vi "Control_Motor_Galil_Hz.vi"() -> ()   [LabVIEW 2015]
uses:
  <vilib>/Instr/_visa.llb/VISA Configure Serial Port (Instr).vi
  <vilib>/regexp/Match Regular Expression.xnode
panel:
  in  "Velocidad":dbl=1.0 format="%#_13g"
  in  "Instrucciones":bool
  in  "No. de Ciclos":dbl=10.0 format="%#_13g"
  in  "Frecuencia":dbl=1.0 format="%#_13g"
  in  "Amplitud":dbl=0.5 format="%#_13g"
  in  "waves 2":bool
  in  "time to save":dbl=0.1
  out "x = y?":bool
  out "GUARDAR":bool
  out "TORQUE":dbl
  out "carga":bool
  out "Boolean 3":bool
  out "whole match":string
  out "size(s)":i32
  out "element":string
  out "x = y? 2":bool
  out "VARIABLE Y":dbl format="%.2f"
  out "VARIABLE X":dbl format="%.2f"
  in  "Combo Box 2":string(combo)="DESPLAZAMIENTO [mm]"
  in  "Combo Box":string(combo)="TIEMPO [s]"
  out "XY Graph":cluster{"TIME SEC":dbl[], "ATT":dbl[]}(graph)
  out "TIME SEC":dbl[](array[numeric]) format="%.2f"
  out "ADD":dbl[](array[numeric]) format="%.2f"
  out "ATT":dbl[](array[numeric]) format="%.2f"
  out "AT":dbl[](array[numeric])
  out "AD":dbl[](array[numeric])
  out "x/y":dbl
  out "result string 2":string
  out "after match":string
  out "result string":string
  out "before match":string
  out "Boolean 2":bool
  out "tiempo [min]":ext
  out "path":path
  out "desplazamiento":dbl format="%.2f"
  out "torque":dbl format="%.2f"
  in  "detener":bool
  in  "VISA resource name":refnum<visa-resource-name>="COM14"
  in  "stop":bool
  in  "bajar":bool
  out "String 2":string
  in  "stop 2":bool
  in  "Filename":path=path "Datos_Motor_Dyn"
  in  "subir":bool
  in  "waves":bool
  in  "Movimiento manual":bool
  out "read buffer":string
  out "return count READ":u32
  out "VARIABLE":string
  out "return count 1":u32
  in  "POSICION":dbl
  out "PULSOS":dbl
  in  "code":string
  out "initialized array":string[](array[string])
  # "EJE X"
  # "EJE Y"
  # "Tiempo adquisición"
  # "Guardando"
  # "[mm/s]"
  # "[mm]"
  # "[Hz]"
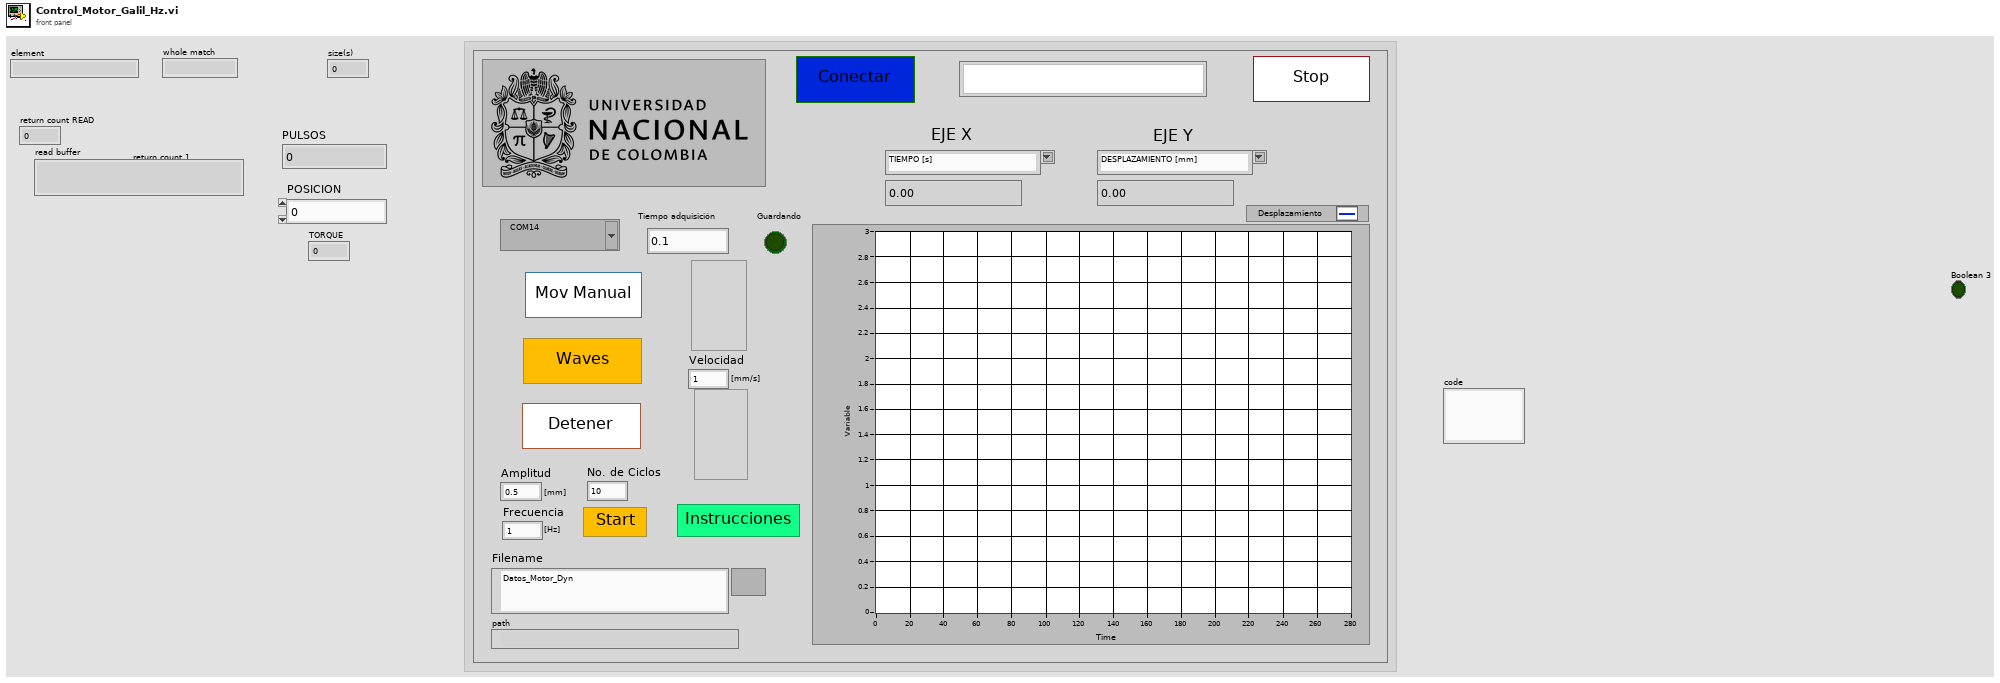
[diagram p1: front panel]
types:
  T1 = enum16{"open", "open or create", "create or replace", "create", "open (read-only)"}
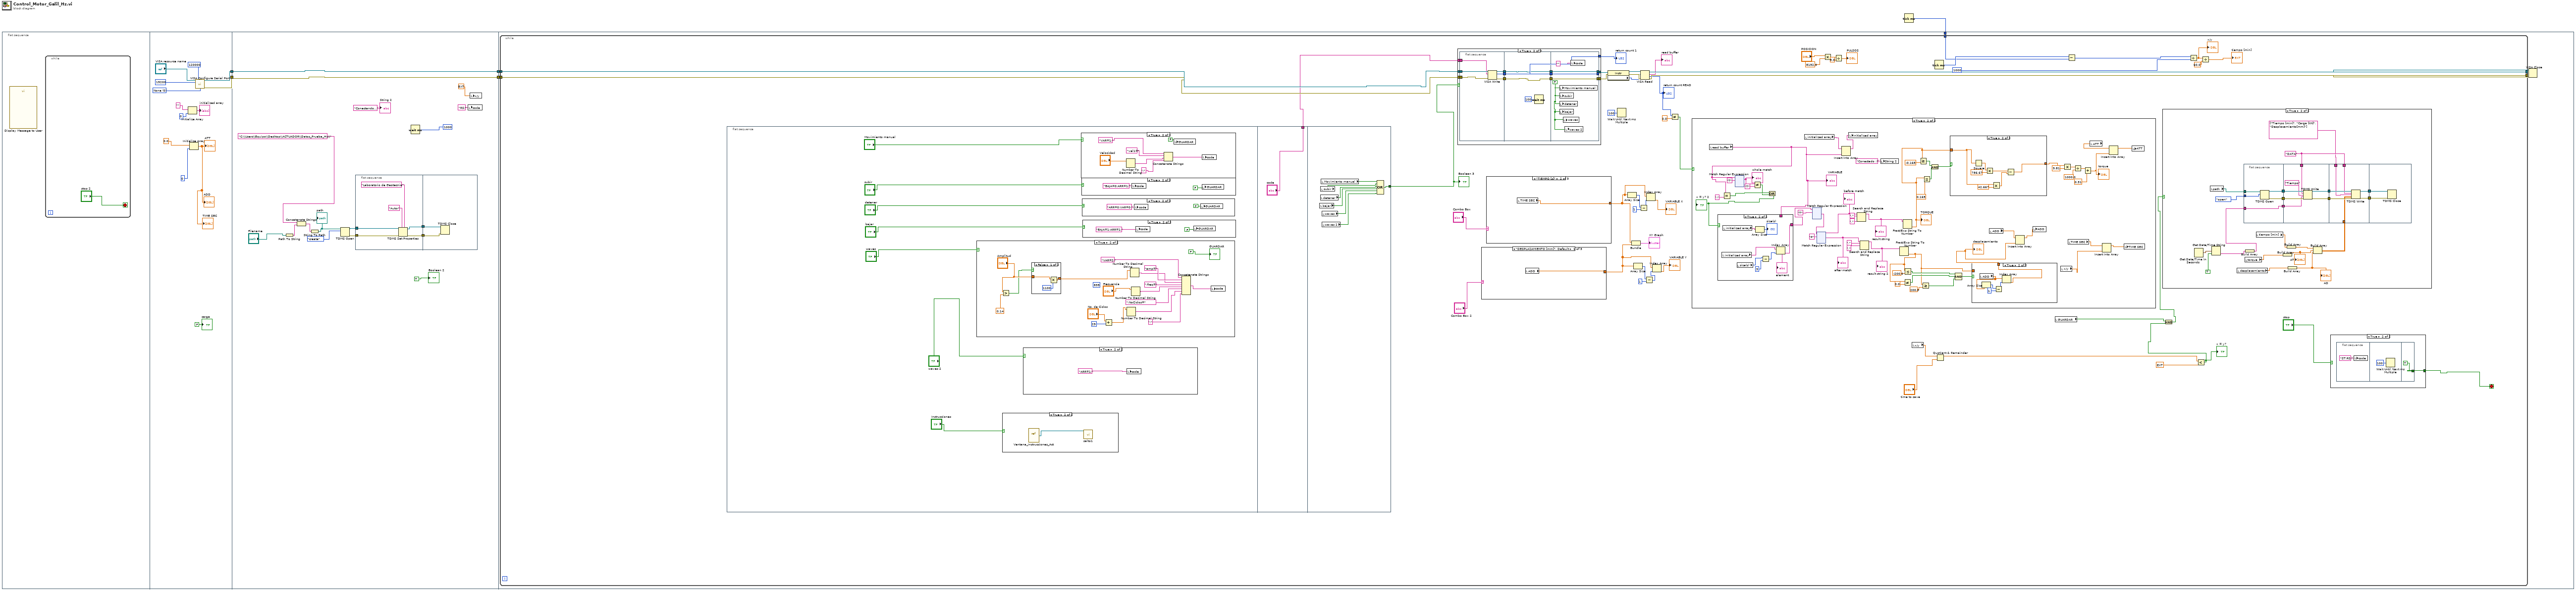
[diagram p0: block diagram]
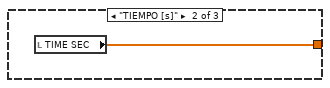
[diagram p3: hidden frame]
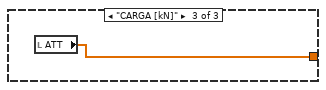
[diagram p4: hidden frame]
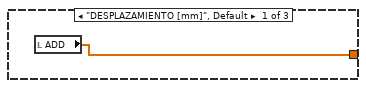
[diagram p5: hidden frame]
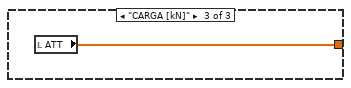
[diagram p6: hidden frame]
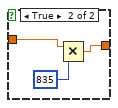
[diagram p11: hidden frame]
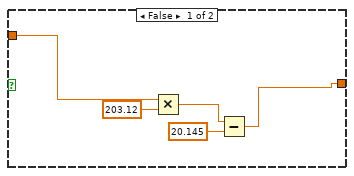
[diagram p19: hidden frame]
diagram:
  n1 = flat-sequence {
    tunnel: [w13] -> w5
    tunnel: [w12] -> w4
    tunnel: [w35] -> w3
    tunnel: [w34] -> w2
    tunnel: w5 -> [w35]
    tunnel: w4 -> [w34]
    tunnel: w3 -> [w49]
    tunnel: w2 -> [w48]
    tunnel: w1 -> [w45]
    frame #0 {
      n2 = call "Display Message to User"() -> ()  [unwired: 10 in, 2 out]
      n3 = while {
        stop <- "stop 2" stop-if-true
      }
    }
    frame #1 {
      w19 = u16 0 items=["None", "XON/XOFF", "RTS/CTS", "XON/XOFF & RTS/CTS", "DTR/DSR", "XON/XOFF & DTR/DSR"] ("flow control (0:none)")
      n4 = Initialize Array("", 0 ("dimension size")) -> (→"initialized array":string[])
      n5 = Initialize Array(0.0, 0 ("dimension size")) -> (→"ATT" →"ADD" →"TIME SEC":dbl[])
      n6 = call-poly "VISA Configure Serial Port"("VISA resource name"="VISA resource name", "timeout (10sec)"=u32 120000, "baud rate (9600)"=u32 19200, "flow control (0:none)"=w19) -> ("VISA resource name out"=w13:refnum<visa-resource-name>, "error out"=w12:errorcluster)  [unwired: 10 in]
      "carga" <- FALSE ("carga")
    }
    frame #2 {
      n7 = Path To String(path="Filename") -> (string=w31:string)
      n8 = Concatenate Strings("C:\\Users\\Equipo\\Desktop\\ACTUADOR\\Datos_Prueba_Hz\\", w31) -> (w30:string)
      n9 = String To Path(string=w30) -> (path=w28:path)
      "path" <- w28
      n10 = TDMS Open(10:T1."create" ("operation (0:open)"), 11:w28) -> (0:w24:errorcluster, 3:w25:refnum<k34>)  [unwired: 5 in]
      n11 = flat-sequence {
        tunnel: [w40] -> w33
        tunnel: [w39] -> w32
        tunnel: w25 -> [w38]
        tunnel: w24 -> [w37]
        tunnel: w33 -> [w44]
        tunnel: w32 -> [w43]
        frame #0 {
          n12 = TDMS Set Properties(5:"Laboratorio de Geotecnia" ("property name"), 7:"Autor" ("property name"), 8:w37, 11:w38) -> (0:w39:errorcluster, 3:w40:refnum<k34>)  [unwired: 2 in, 2 out]
        }
        frame #1 {
          n13 = TDMS Close(8:w43, 11:w44) -> ()  [unwired: 2 out]
        }
      }
      n14 = Wait (ms)(milliseconds to wait=u32 1000) -> ()  [unwired: 1 out]
      n15 = local write "code"("RS;" ("code")) -> ()
      n16 = local write "x/y"(ext 0.0 ("x-y*floor(x/y)")) -> ()
      "String 2" <- "Conectando..." ("String 2")
      "Boolean 2" <- TRUE
    }
    frame #3 {
      n17 = while {
        tunnel: w49 -> [w89]
        tunnel: w48 -> [w88]
        tunnel: [w96] -> w47
        tunnel: [w95] -> w46
        tunnel: w45 -> [w72]
        stop <- w58 stop-if-true
        n18 = flat-sequence {
          tunnel: ["code"] -> w79
          tunnel: [w202] -> w80
          frame #0 {
            n19 = case shown="True" "waves" {
              frame False {
              }
              frame True {
                (unwired) 835
                n20 = Greater?(x="Amplitud", y=0.14) -> (0:w163:bool)
                n21 = case shown="False" w163 {
                  tunnel: [w181 w185] -> w166
                  tunnel: "Amplitud" -> [w182 w184]
                  frame False {
                    n22 = Multiply(x=w182, y=1100) -> (x*y=w181:dbl)
                  }
                  frame True {
                    n23 = Multiply(x=w184, y=835) -> (x*y=w185:dbl)
                  }
                }
                n24 = Add(x="No. de Ciclos", y=29) -> (x+y=w171:dbl)
                n25 = Number To Decimal String(number=w171) -> (decimal integer string=w173:string)  [unwired: 1 in]
                n26 = Number To Decimal String(number=w166) -> (decimal integer string=w177:string)  [unwired: 1 in]
                n27 = Number To Decimal String(number="Frecuencia") -> (decimal integer string=w167:string)  [unwired: 1 in]
                n28 = Concatenate Strings("VAR=2;" ("code"), "amp=", w177, ";freq=", w167, ";NoCiclos=", w173, ";") -> (w174:string)
                n29 = local write "code"(w174) -> ()
                "GUARDAR" <- FALSE
              }
            }
            n30 = case shown="True" "Instrucciones" {
              frame False {
              }
              frame True {
                n31 = vi-ref "Ventana_Instrucciones_Act.vi"() -> (w161:refnum<vi>)
                n32 = call "salto1.vi"("reference"=w161) -> ()  [unwired: 15 in]
              }
            }
            n33 = case shown="True" "waves 2" {
              frame False {
              }
              frame True {
                n34 = local write "code"("ARR=1;" ("code")) -> ()
              }
            }
            n35 = case shown="True" "Movimiento manual" {
              frame False {
              }
              frame True {
                n36 = Number To Decimal String(number="Velocidad") -> (decimal integer string=w194:string)  [unwired: 1 in]
                n37 = Concatenate Strings("VAR=1;" ("code"), "vel1=", w194, ";") -> (w197:string)
                n38 = local write "GUARDAR"(FALSE) -> ()
                n39 = local write "code"(w197) -> ()
              }
            }
            n40 = case shown="True" "subir" {
              frame False {
              }
              frame True {
                n41 = local write "code"("BAJA=0;ARR=1;" ("code")) -> ()
                n42 = local write "GUARDAR"(FALSE ("GUARDAR")) -> ()
              }
            }
            n43 = case shown="True" "detener" {
              frame False {
              }
              frame True {
                n44 = local write "code"("ARR=0;VAR=0;" ("code")) -> ()
                n45 = local write "GUARDAR"(FALSE ("GUARDAR")) -> ()
              }
            }
            n46 = case shown="True" "bajar" {
              frame False {
              }
              frame True {
                n47 = local write "code"("BAJA=1;ARR=1;" ("code")) -> ()
                n48 = local write "GUARDAR"(FALSE ("GUARDAR")) -> ()
              }
            }
          }
          frame #1 {
          }
          frame #2 {
            n49 = local read "bajar"() -> (w206:bool)
            n50 = local read "detener"() -> (w205:bool)
            n51 = local read "subir"() -> (w204:bool)
            n52 = local read "Movimiento manual"() -> (w203:bool)
            n53 = local read "waves"() -> (w207:bool)
            n54 = local read "waves 2"() -> (w201:bool)
            n55 = Compound Arithmetic op=OR(w203, w204, w205, w206, w207, w201) -> (w202:bool)
          }
        }
        n56 = case shown="True" w80 {
          tunnel: w89 -> [w629 w638]
          tunnel: w88 -> [w628 w637]
          tunnel: [w629 w636] -> w90
          tunnel: [w628 w635] -> w100
          tunnel: w79 -> [_ w634]
          tunnel: [_ w633] -> w87
          frame False {
          }
          frame True {
            n57 = flat-sequence {
              tunnel: w638 -> [w647]
              tunnel: w637 -> [w646]
              tunnel: [w645] -> w641
              tunnel: [w644] -> w640
              tunnel: [w643] -> w639
              tunnel: w634 -> [w642]
              tunnel: w641 -> [w649]
              tunnel: w640 -> [w648]
              tunnel: w639 -> [w651]
              tunnel: [w649] -> w632
              tunnel: [w648] -> w631
              tunnel: [w651] -> w630
              tunnel: [w654] -> w633
              tunnel: [w655] -> w635
              tunnel: [w656] -> w636
              tunnel: w632 -> [w656]
              tunnel: w631 -> [w655]
              tunnel: w630 -> [w654]
              frame #0 {
                n58 = VISA Write(VISA resource name=w647, write buffer=w642, error in (no error)=w646) -> (VISA resource name out=w645:refnum<visa-resource-name>, return count=w643:u32, error out=w644:errorcluster)
              }
              frame #1 {
                n59 = Wait (ms)(milliseconds to wait=u32 100) -> ()  [unwired: 1 out]
              }
              frame #2 {
                w652 = FALSE
                n60 = local write "Movimiento manual"(w652) -> ()
                n61 = local write "subir"(w652) -> ()
                n62 = local write "detener"(w652) -> ()
                n63 = local write "bajar"(w652) -> ()
                n64 = local write "waves"(w652) -> ()
                n65 = local write "waves 2"(w652) -> ()
                n66 = local write "code"("" ("code")) -> ()
              }
            }
          }
        }
        "return count 1" <- w87
        n67 = case shown="\"DESPLAZAMIENTO [mm]\", Default" "Combo Box 2" {
          tunnel: [w105 w106 w107] -> w65
          frame "DESPLAZAMIENTO [mm]", Default {
            n68 = local read "ADD"() -> (w105:dbl[])
          }
          frame "TIEMPO [s]" {
            n69 = local read "TIME SEC"() -> (w106:dbl[])
          }
          frame "CARGA [kN]" {
            n70 = local read "ATT"() -> (w107:dbl[])
          }
        }
        n71 = case shown="\"TIEMPO [s]\"" "Combo Box" {
          tunnel: [w108 w109 w110] -> w67
          frame "DESPLAZAMIENTO [mm]", Default {
            n72 = local read "ADD"() -> (w108:dbl[])
          }
          frame "TIEMPO [s]" {
            n73 = local read "TIME SEC"() -> (w109:dbl[])
          }
          frame "CARGA [kN]" {
            n74 = local read "ATT"() -> (w110:dbl[])
          }
        }
        n75 = property class="Instr"(reference=w90, error in=w100) -> (reference out=w99:refnum<visa-resource-name>, error out=w98:errorcluster, "Serial Settings:Number of Bytes at Serial Port"=w97:u32)
        n76 = Wait Until Next ms Multiple(millisecond multiple=u32 100) -> ()  [unwired: 1 out]
        n77 = Array Size(array=w67) -> (size(s)=w61:i32)
        n78 = Bundle("ATT"=w67, "ATT"=w65) -> (→"XY Graph":cluster{"ATT":dbl[], "ATT":dbl[]})  [unwired: 1 in]
        n79 = Array Size(array=w65) -> (size(s)=w64:i32)
        n80 = Subtract(x=w61, y=1) -> (x-y=w60:i32)
        n81 = VISA Read(VISA resource name=w99, byte count=w97, error in (no error)=w98) -> (VISA resource name out=w96:refnum<visa-resource-name>, read buffer=→"read buffer":string, return count=w91:u32, error out=w95:errorcluster)
        "return count READ" <- w91
        n82 = Subtract(x=w64, y=1) -> (x-y=w63:i32)
        n83 = Index Array(array=w67, index=w60) -> (element=→"VARIABLE X":dbl)
        n84 = Index Array(array=w65, index=w63) -> (element=→"VARIABLE Y":dbl)
        n85 = Not Equal?(x=w91, y=0.0) -> (x != y?=w93:bool)
        n86 = case shown="True" w93 {
          frame False {
          }
          frame True {
            n87 = local read "read buffer"() -> (w226:string)
            "VARIABLE" <- w226
            n88 = Equal?(x=w226, y=":") -> (x = y?=w224:bool)
            n89 = xnode "Match Regular Expression"("input string"=w226, "regular expression"="T") -> ("whole match"=w222:string)  [unwired: 4 in, 4 out]
            "whole match" <- w222
            n90 = Not Equal?(x=w222, y="T") -> (x != y?=w220:bool)
            n91 = Or(x=w224, y=w220) -> (x .or. y?=w223:bool)
            "x = y? 2" <- w223
            n92 = case shown="True" w223 {
              tunnel: [w380 w387] -> w227
              tunnel: w226 -> [w380 _]
              frame False {
              }
              frame True {
                n93 = local read "initialized array"() -> (w386:string[])
                n94 = local read "initialized array"() -> (w385:string[])
                n95 = local read "size(s)"() -> (w383:i32)
                n96 = Array Size(array=w385) -> (size(s)=→"size(s)":i32)
                n97 = Subtract(x=w383, y=3) -> (x-y=w381:i32)
                n98 = Index Array(array=w386, index=w381) -> (element=w387:string)
                "element" <- w387
              }
            }
            n99 = local read "initialized array"() -> (w258:string[])
            n100 = xnode "Match Regular Expression"("input string"=w227, "regular expression"="T") -> ("after match"=w254:string)  [unwired: 4 in, 4 out]
            n101 = xnode "Match Regular Expression"("input string"=w254, "regular expression"="P") -> ("before match"=w253:string, "after match"=w247:string)  [unwired: 4 in, 3 out]
            "before match" <- w253
            "after match" <- w247
            n102 = Insert Into Array(array=w258, new element=w226) -> (w259:string[])  [unwired: 1 in]
            n103 = local write "initialized array"(w259) -> ()
            n104 = Search and Replace String(input string=w253, search string=".", replace string="," ("replace string (\"\")")) -> (result string=w250:string)  [unwired: 5 in, 3 out]
            "result string" <- w250
            n105 = Search and Replace String(input string=w247, search string=".", replace string="," ("replace string (\"\")")) -> (result string=w248:string)  [unwired: 5 in, 3 out]
            "result string 2" <- w248
            n106 = local write "String 2"("Conectado :)" ("String 2")) -> ()
            n107 = Fract/Exp String To Number(string=w248) -> (number=w213:dbl)  [unwired: 3 in, 1 out]
            n108 = Fract/Exp String To Number(string=w250) -> (number=w233:dbl)  [unwired: 3 in, 1 out]
            "TORQUE" <- w233
            n109 = Not Equal?(x=w213, y=0.0) -> (x != y?=w217:bool)
            n110 = Less Or Equal?(x=w213, y=-200.0) -> (x <= y?=w218:bool)
            n111 = Greater Or Equal?(x=w233, y=-0.165) -> (x >= y?=w236:bool)
            n112 = Greater Or Equal?(x=w213, y=200.0) -> (x >= y?=w216:bool)
            n113 = Less Or Equal?(x=w233, y=0.165) -> (x <= y?=w237:bool)
            n114 = And(x=w236, y=w237) -> (x .and. y?=w238:bool)
            n115 = case shown="True" w238 {
              tunnel: w233 -> [w392 w396]
              tunnel: [w388 w393] -> w232
              frame False {
                n116 = Multiply(x=w392, y=203.12) -> (x*y=w390:dbl)
                n117 = Subtract(x=w390, y=20.145) -> (x-y=w388:dbl)
              }
              frame True {
                n118 = Square(x=w396) -> (x^2=w399:dbl)
                n119 = Multiply(x=w399, y=786.67) -> (x*y=w397:dbl)
                n120 = Multiply(x=w396, y=42.667) -> (x*y=w394:dbl)
                n121 = Subtract(x=w397, y=w394) -> (x-y=w393:dbl)
              }
            }
            n122 = Compound Arithmetic op=AND(w218, w217, w216) -> (w211:bool)
            n123 = case shown="True" w211 {
              tunnel: [w260 w261] -> w212
              tunnel: w213 -> [w260 _]
              frame False {
              }
              frame True {
                n124 = local read "ADD"() -> (w265:dbl[])
                n125 = Array Size(array=w265) -> (size(s)=w264:i32)
                n126 = Subtract(x=w264, y=1) -> (x-y=w263:i32)
                n127 = Index Array(array=w265, index=w263) -> (element=w261:dbl)
              }
            }
            "desplazamiento" <- w212
            n128 = local read "ADD"() -> (w242:dbl[])
            n129 = Insert Into Array(array=w242, new element=w212) -> (w243:dbl[])  [unwired: 1 in]
            n130 = local write "ADD"(w243) -> ()
            n131 = local read "x/y"() -> (w239:dbl)
            n132 = Multiply(x=w232, y=9.81) -> (x*y=w230:dbl)
            n133 = local read "TIME SEC"() -> (w240:dbl[])
            n134 = Divide(x=w230, y=1000.0) -> (x/y=w210:dbl)
            n135 = Add(x=w210, y=0.31) -> (x+y=w208:dbl)
            "torque" <- w208
            n136 = local read "ATT"() -> (w245:dbl[])
            n137 = Insert Into Array(array=w240, new element=w239) -> (w241:dbl[])  [unwired: 1 in]
            n138 = Insert Into Array(array=w245, new element=w208) -> (w244:dbl[])  [unwired: 1 in]
            n139 = local write "TIME SEC"(w241) -> ()
            n140 = local write "ATT"(w244) -> ()
          }
        }
        n141 = Multiply(x="POSICION", y=8192.0) -> (x*y=w83:dbl)
        n142 = Divide(x=w83, y=5.0) -> (x/y=→"PULSOS":dbl)
        n143 = local read "x/y"() -> (w55:dbl)
        n144 = Tick Count (ms)() -> (millisecond timer value=w78:u32)
        n145 = Quotient & Remainder(x=w55, y="time to save") -> (x-y*floor(x/y)=w51:dbl)  [unwired: 1 out]
        n146 = local read "GUARDAR"() -> (w54:bool)
        n147 = Subtract(x=w78, y=w72) -> (x-y=w77:u32)
        n148 = Divide(x=w77, y=u32 1000) -> (x/y=w75:dbl)
        "x/y" <- w75
        n149 = Less?(x=w51, y=ext 0.05) -> (x < y?=w52:bool)
        "x = y?" <- w52
        n150 = And(x=w54, y=w52) -> (x .and. y?=w53:bool)
        n151 = case shown="True" w53 {
          frame False {
          }
          frame True {
            w121 = "DATA"
            n152 = Get Date/Time In Seconds() -> (seconds since 1Jan1904=w123:timestamp)
            n153 = local read "path"() -> (w125:path)
            n154 = Get Date/Time String(seconds (now)=w123, want seconds? (F)=TRUE) -> (time string=w111:string)  [unwired: 1 in, 1 out]
            n155 = local read "desplazamiento"() -> (w114:dbl)
            n156 = flat-sequence {
              tunnel: w125 -> [w137]
              tunnel: [w136] -> w132
              tunnel: [w135] -> w131
              tunnel: w122 -> [w134]
              tunnel: [w134] -> w130
              tunnel: T1."open" ("operation (0:open)") -> [w133]
              tunnel: w132 -> [w144]
              tunnel: [w143] -> w129
              tunnel: w131 -> [w142]
              tunnel: [w141] -> w128
              tunnel: w130 -> [w140]
              tunnel: w121 -> [w139]
              tunnel: w129 -> [w151]
              tunnel: w128 -> [w150]
              tunnel: w121 -> [w149]
              tunnel: string[] ["Tiempo [min]", "Carga [kN]", "Desplazamiento[mm]"] ("channel name(s) in (Untitled)") -> [w148]
              tunnel: [w147] -> w127
              tunnel: [w146] -> w126
              tunnel: w117 -> [w145]
              tunnel: w127 -> [w153]
              tunnel: w126 -> [w152]
              frame #0 {
                n157 = TDMS Open(10:w133, 11:w137) -> (0:w135:errorcluster, 3:w136:refnum<k34>)  [unwired: 5 in]
              }
              frame #1 {
                n158 = TDMS Write(0:w144, 5:w139, 7:"Tiempo" ("channel name(s) in (Untitled)"), 9:w140, 11:w142) -> (4:w143:refnum<k34>, 15:w141:errorcluster)  [unwired: 1 in, 2 out]
              }
              frame #2 {
                n159 = TDMS Write(0:w151, 5:w149, 7:w148, 9:w145, 11:w150) -> (4:w146:refnum<k34>, 15:w147:errorcluster)  [unwired: 1 in, 2 out]
              }
              frame #3 {
                n160 = TDMS Close(8:w153, 11:w152) -> ()  [unwired: 2 out]
              }
            }
            n161 = local read "torque"() -> (w113:dbl)
            n162 = Build Array(w111) -> (w122:string[])
            n163 = local read "tiempo [min]"() -> (w115:ext)
            n164 = Build Array(w113) -> (w118:dbl[])
            "AT" <- w118
            n165 = Build Array(w115) -> (w119:ext[])
            n166 = Build Array(w114) -> (w116:dbl[])
            "AD" <- w116
            n167 = Build Array(w119, w118, w116) -> (w117:ext[][])
          }
        }
        n168 = Divide(x=w75, y=60.0) -> (x/y=→"tiempo [min]":dbl)
        n169 = case shown="True" "stop" {
          tunnel: [_ w101] -> w58
          frame False {
          }
          frame True {
            n170 = flat-sequence {
              tunnel: [TRUE] -> w101
              frame #0 {
                n171 = local write "code"("ST;RS;" ("code")) -> ()
              }
              frame #1 {
                n172 = Wait Until Next ms Multiple(millisecond multiple=u32 100) -> ()  [unwired: 1 out]
              }
              frame #2 {
              }
            }
          }
        }
        "Boolean 3" <- w80
      }
      n173 = VISA Close(VISA resource name=w47, error in (no error)=w46) -> ()  [unwired: 1 out]
    }
  }
  n174 = Tick Count (ms)() -> (millisecond timer value=w1:u32)
